vi "AIM 664 test Deployment Disabled Custom Device.vi"(8 "error in":errorcluster, 11 "reference in":refnum<class "AIM_Deployment.lvclass">) -> (0 "error out":errorcluster, 3 "reference out":refnum<class "AIM_Deployment.lvclass">)   [LabVIEW 2020, in "AIM_Deployment.lvclass"]
uses:
  AIM_Deployment.lvclass
  <vilib>/addons/_JKI Toolkits/VI Tester/TestCase.llb/TestCase.lvclass
  <vilib>/NI/VeriStand Custom Device Testing Tools/VeriStandTestUtilities/VeriStandTestUtilities.lvlib
  297c49c7-5231-4abd-9dfa-9525516e01de.vi
  Scripting/AIM ARINC 664 Scripting.lvlib
  C:/Program Files (x86)/National Instruments/LabVIEW 2020/vi.lib/NI/VeriStand Custom Device Testing Tools/VeriStandTestCase/VeriStandTestCase.lvclass
  C:/Program Files (x86)/National Instruments/LabVIEW 2020/vi.lib/addons/_JKI Toolkits/VI Tester/TestCase.llb/TestCase.lvclass
  C:/repos/niveristand-aim-arinc664-custom-device/Source/Custom Device Support/Tests/System/AIM_Deployment/AIM_Deployment.lvclass
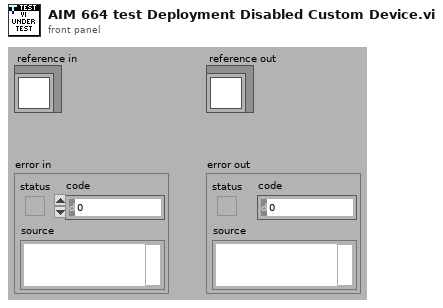
[diagram p1: front panel]
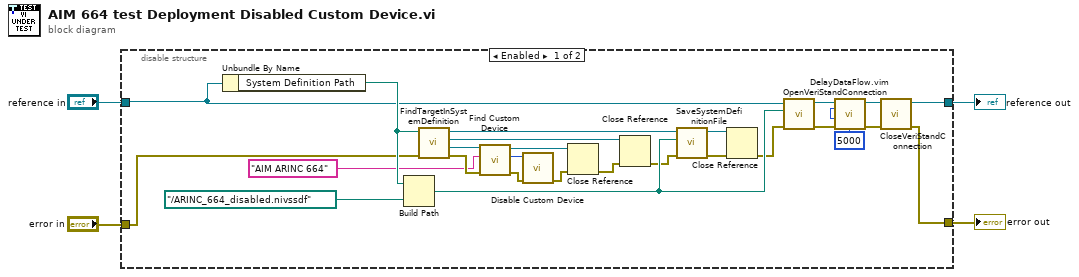
[diagram p0: block diagram]
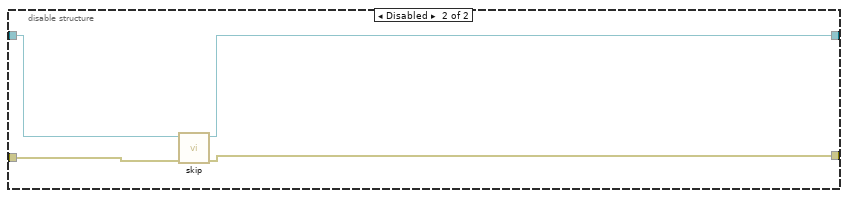
[diagram p2: hidden frame]
diagram:
  n1 = disable-structure shown="Enabled" {
    disable-tunnel: "reference in" -> [w8 w33]
    disable-tunnel: "error in" -> [w7 w32]
    disable-tunnel: [w5 w31] -> w2
    disable-tunnel: [w6 w30] -> w1
    frame Enabled {
      n2 = Unbundle By Name(w8) -> ("System Definition Path"=w21:path)
      n3 = Build Path(base path=w21, name or relative path=path "../ARINC_664_disabled.nivssdf") -> (appended path=w29:path)
      n4 = call <vilib>:"FindTargetInSystemDefinition.vi"("error in"=w7, "system definition path"=w21) -> ("error out"=w23:errorcluster, "Target"=w22:refnum<k24>, "Root"=w17:refnum<k24>, "System Definition"=w20:refnum<k24>)  [unwired: 6 in]
      n5 = call "Find Custom Device.vi"("error in"=w23, "name"="AIM ARINC 664" ("custom device name"), "target in"=w22) -> ("error out"=w25:errorcluster, "custom device"=w24:u64, "target out"=w27:refnum<k24>)  [unwired: 6 in]
      n6 = call "Disable Custom Device.vi"("error in"=w25, "custom device ref in"=w24) -> ("error out"=w26:errorcluster)  [unwired: 8 in, 1 out]
      n7 = Close Reference(reference=w27, error in (no error)=w26) -> (error out=w15:errorcluster)
      n8 = Close Reference(reference=w17, error in (no error)=w15) -> (error out=w16:errorcluster)
      n9 = call <vilib>:"SaveSystemDefinitionFile.vi"("error in (no error)"=w16, "System Definition File in"=w29, "System Definition Reference in"=w20) -> ("error out"=w18:errorcluster, "System Definition Reference out"=w19:refnum<k24>)  [unwired: 7 in]
      n10 = Close Reference(reference=w19, error in (no error)=w18) -> (error out=w28:errorcluster)
      n11 = call-dynamic "OpenVeriStandConnection.vi"("error in (no error)"=w28, "System Definition File"=w29, "VeriStand Test Case in"=w8) -> ("error out"=w12:errorcluster, "VeriStand Test Case out"=w14:refnum<class "AIM_Deployment.lvclass">)  [unwired: 6 in, 1 out]
      n12 = call "DelayDataFlow.vim"("value in"=w12, "milliseconds to wait"=u32 5000) -> ("value out"=w13:errorcluster)  [unwired: 2 in, 1 out]
      n13 = call-dynamic "CloseVeriStandConnection.vi"("error in (no error)"=w13, "VeriStand Test Case in"=w14) -> ("error out"=w5:errorcluster, "VeriStand Test Case out"=w6:refnum<class "AIM_Deployment.lvclass">)  [unwired: 8 in]
    }
    frame Disabled {
      n14 = call <vilib>:"skip.vi"("error in (no error)"=w32, "TestCase in"=w33) -> ("error out"=w31:errorcluster, "TestCase out"=w30:refnum<class "AIM_Deployment.lvclass">)  [unwired: 8 in]
    }
  }
  "error out" <- w2
  "reference out" <- w1
